vi "Pulse generator2.vi"(2 "Framedur":i32=1000, 3 "duty cylcle":dbl=0.5, 4 "error in":errorcluster, 5 "Counter freq":u16=200) -> (0 "error out":errorcluster, 1 "# of pulses":i32)   [LabVIEW 2013]
uses:
  <vilib>/DAQmx/create/channels.llb/DAQmx Create Channel (CI-Count Edges).vi
  <vilib>/DAQmx/create/channels.llb/DAQmx Create Channel (CO-Pulse Generation-Frequency).vi
  <vilib>/DAQmx/configure/timing.llb/DAQmx Timing (Implicit).vi
  <vilib>/DAQmx/configure/trigger.llb/DAQmx Start Trigger (Digital Edge).vi
  Global 1.vi
  <vilib>/DAQmx/read.llb/DAQmx Read (Counter U32 1Chan 1Samp).vi
  <resource>/objmgr/daqmx.rc
panel:
  in  "stop":bool
  in  "Counter":tag="Dev1/ctr1"
  in  "Input Terminal":tag="/Dev1/PFI1"
  in  "counter":tag="Dev1/ctr0"
  in  "CTR Trigger":tag="/Dev1/PFI0"
  in  "initial delay":dbl format="%.6f"
  # "This counter is for generating pulses."
  # "This counter is for counting the number of pulses that the counter above generated."
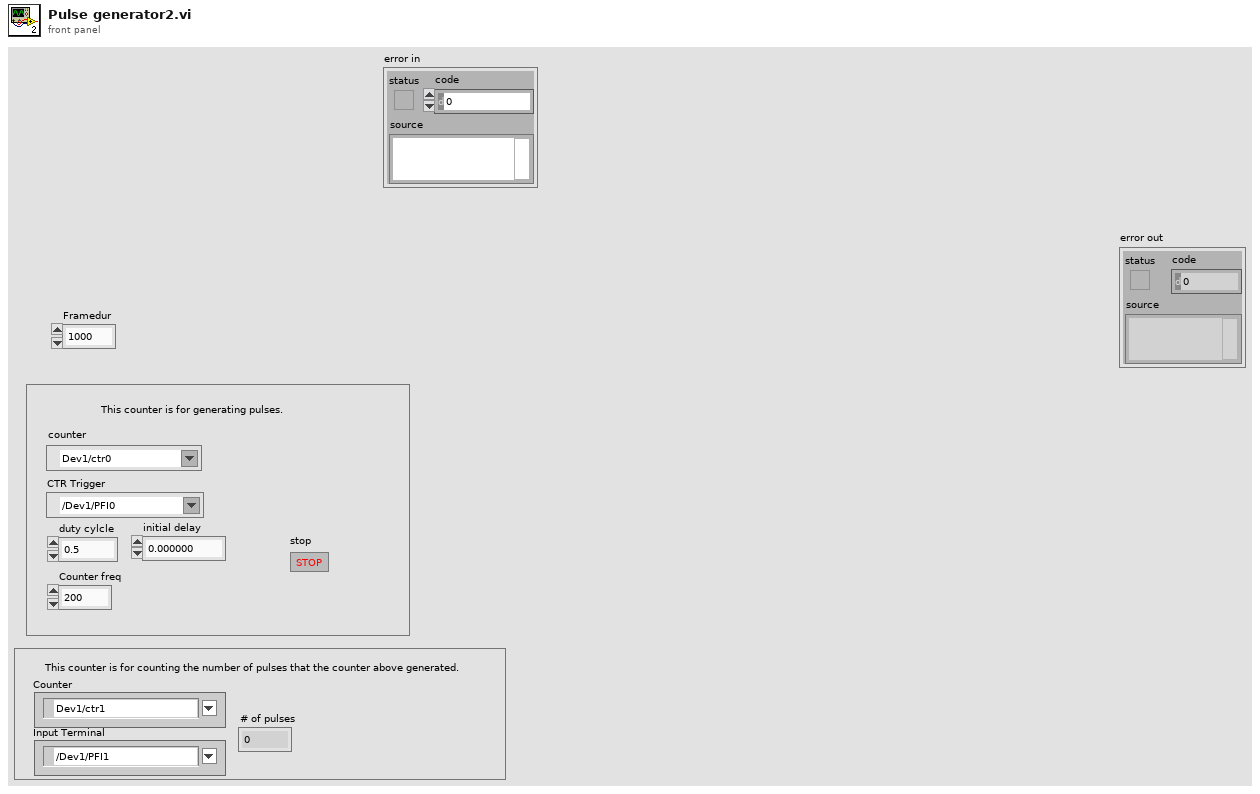
[diagram p1: front panel]
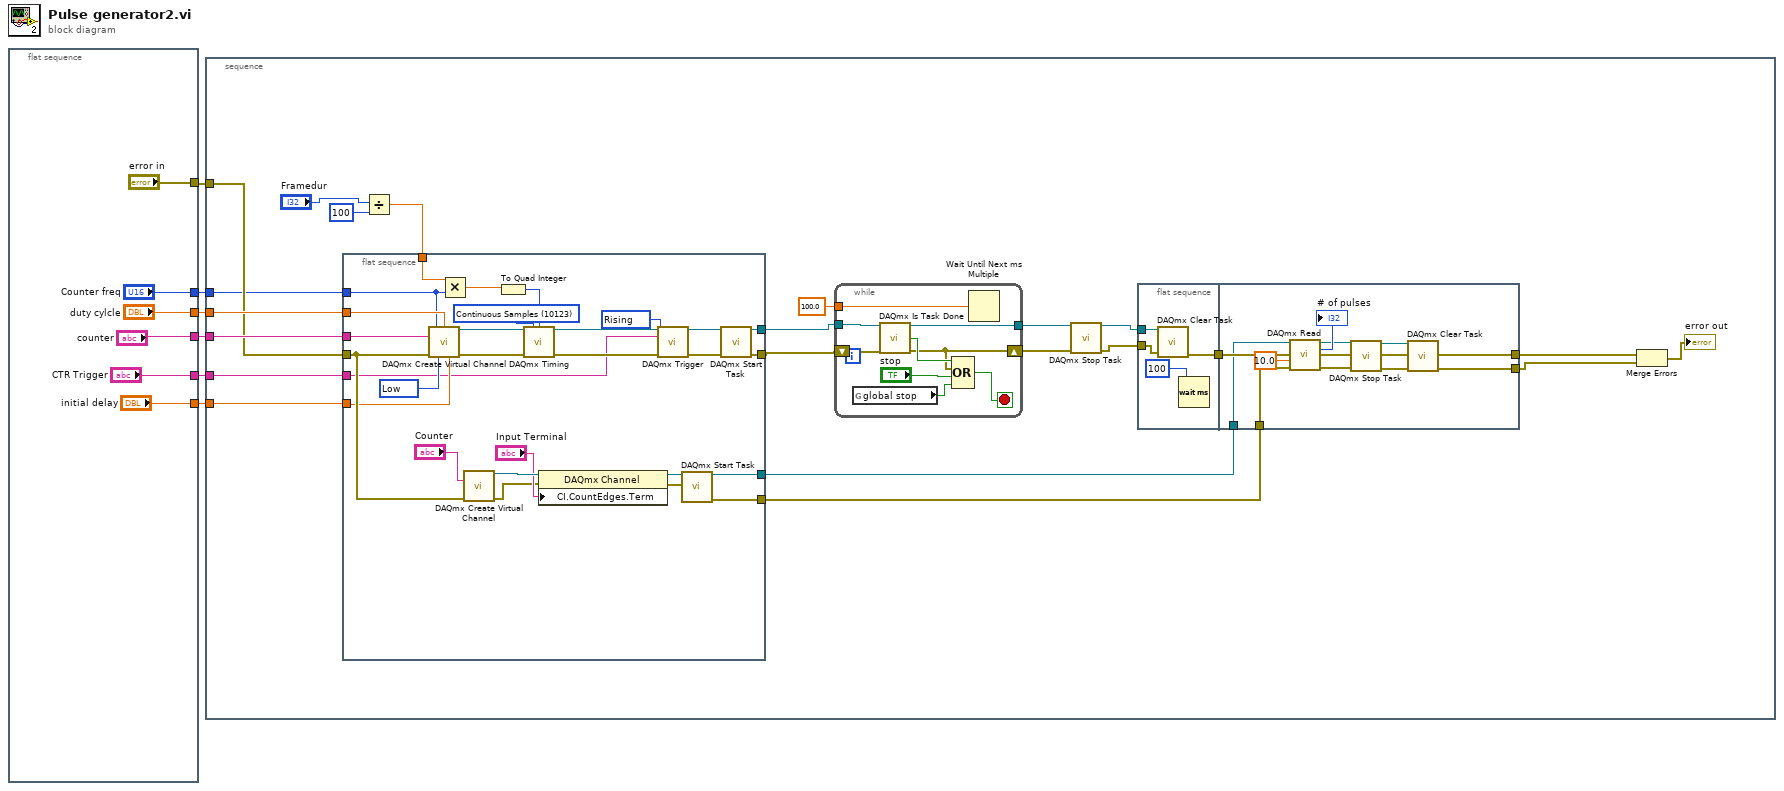
[diagram p0: block diagram]
diagram:
  n1 = flat-sequence {
    tunnel: ["counter"] -> w6
    tunnel: ["duty cylcle"] -> w5
    tunnel: ["error in"] -> w4
    tunnel: ["CTR Trigger"] -> w3
    tunnel: ["Counter freq"] -> w2
    tunnel: ["initial delay"] -> w1
    frame #0 {
    }
  }
  n2 = stacked-sequence {
    tunnel: w6 -> [w34]
    tunnel: w4 -> [w30]
    tunnel: w5 -> [w33]
    tunnel: w3 -> [w25]
    tunnel: w2 -> [w24]
    tunnel: w1 -> [w23]
    frame #0 {
      n3 = flat-sequence {
        tunnel: w34 -> [w64]
        tunnel: w33 -> [w61]
        tunnel: w20 -> [w60]
        tunnel: [w58] -> w18
        tunnel: [w57] -> w19
        tunnel: w30 -> [w48]
        tunnel: [w50] -> w28
        tunnel: [w49] -> w27
        tunnel: w25 -> [w44]
        tunnel: w24 -> [w47]
        tunnel: w23 -> [w46]
        frame #0 {
          w45 = 10280 items=["Rising"=10280, "Falling"=10171] ("edge")
          w59 = 10214 items=["High"=10192, "Low"=10214] ("idle state")
          w69 = 10123 items=["Finite Samples"=10178, "Continuous Samples"=10123, "Hardware Timed Single Point"=12522] ("sample mode")
          n4 = call-poly <vilib>:"DAQmx Create Virtual Channel.vi"("frequency"=w47, "duty cycle"=w61, "counter"=w64, "error in"=w48, "idle state"=w59, "initial delay"=w46) -> ("task out"=w70:refnum<k21>, "error out"=w71:errorcluster)  [unwired: 8 in]
          n5 = Multiply(x=w60, y=w47) -> (x*y=w63:dbl)
          n6 = call-poly <vilib>:"DAQmx Create Virtual Channel.vi"("counter"="Counter", "error in"=w48) -> ("task out"=w55:refnum<k21>, "error out"=w53:errorcluster)  [unwired: 12 in]
          n7 = To Quad Integer(1:w63) -> (0:w62:i64)
          n8 = call-poly <vilib>:"DAQmx Timing.vi"("task/channels in"=w70, "sample mode"=w69, "samples per channel"=w62, "error in"=w71) -> ("task out"=w67:refnum<k21>, "error out"=w68:errorcluster)  [unwired: 10 in]
          n9 = property class="DAQmx Channel"(reference=w55, error in=w53, "CI.CountEdges.Term"="Input Terminal") -> (reference out=w52:refnum<k21>, error out=w51:errorcluster)
          n10 = call-poly <vilib>:"DAQmx Trigger.vi"("task/channels in"=w67, "source"=w44, "edge"=w45, "error in"=w68) -> ("task out"=w65:refnum<k21>, "error out"=w66:errorcluster)  [unwired: 10 in]
          n11 = call <vilib>:"DAQmx Start Task.vi"("task/channels in"=w52, "error in"=w51) -> ("task out"=w50:refnum<k21>, "error out"=w49:errorcluster)  [unwired: 12 in]
          n12 = call <vilib>:"DAQmx Start Task.vi"("task/channels in"=w65, "error in"=w66) -> ("task out"=w58:refnum<k21>, "error out"=w57:errorcluster)  [unwired: 12 in]
        }
      }
      n13 = Divide(x="Framedur", y=100) -> (x/y=w20:dbl)
      n14 = while {
        tunnel: w18 -> [w43]
        shift-right: [w38] -> w13
        shift-left: w19 -> [w42]
        tunnel: [w41] -> w16
        tunnel: sgl 100.0 ("millisecond multiple") -> [w40]
        stop <- w37 stop-if-true
        n15 = global read "Global 1.vi" "global stop"() -> (w36:bool)
        n16 = call <vilib>:"DAQmx Is Task Done.vi"("task/channels in"=w43, "error in"=w42) -> ("task out"=w41:refnum<k21>, "task done?"=w39:bool, "error out"=w38:errorcluster)  [unwired: 11 in]
        n17 = Compound Arithmetic op=OR(w39, w38, "stop", w36) -> (w37:bool)
        n18 = Wait Until Next ms Multiple(millisecond multiple=w40) -> ()  [unwired: 1 out]
      }
      n19 = call <vilib>:"DAQmx Stop Task.vi"("task/channels in"=w16, "error in"=w13) -> ("task out"=w15:refnum<k21>, "error out"=w14:errorcluster)  [unwired: 12 in]
      n20 = flat-sequence {
        tunnel: [w75] -> w29
        tunnel: w15 -> [w73]
        tunnel: w14 -> [w72]
        tunnel: [w85] -> w32
        tunnel: w29 -> [w85]
        tunnel: w28 -> [w78]
        tunnel: w27 -> [w77]
        tunnel: [w76] -> w26
        frame #0 {
          n21 = call <vilib>:"DAQmx Clear Task.vi"("task in"=w73, "error in"=w72) -> ("error out"=w75:errorcluster)  [unwired: 13 in]
          n22 = Wait (ms)(milliseconds to wait=u32 100) -> ()  [unwired: 1 out]
        }
        frame #1 {
          n23 = call-poly <vilib>:"DAQmx Read.vi"("task/channels in"=w78, "timeout"=10.0, "error in"=w77) -> ("task out"=w81:refnum<k21>, "data"=→"# of pulses":u32, "error out"=w82:errorcluster)  [unwired: 10 in]
          n24 = call <vilib>:"DAQmx Stop Task.vi"("task/channels in"=w81, "error in"=w82) -> ("task out"=w79:refnum<k21>, "error out"=w80:errorcluster)  [unwired: 12 in]
          n25 = call <vilib>:"DAQmx Clear Task.vi"("task in"=w79, "error in"=w80) -> ("error out"=w76:errorcluster)  [unwired: 13 in]
        }
      }
      n26 = Merge Errors(w32, w26) -> (→"error out":errorcluster)
    }
  }
